vi "AMVoltsordB.vi"(8 "Min Power":dbl=10.0, 9 "Peak Power":dbl=20.0, 10 "Signal In":dbl, 11 "Linear?":bool) -> (2 "Out":dbl)   [LabVIEW 2012]
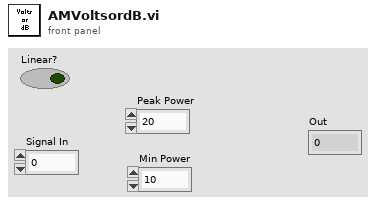
[diagram p1: front panel]
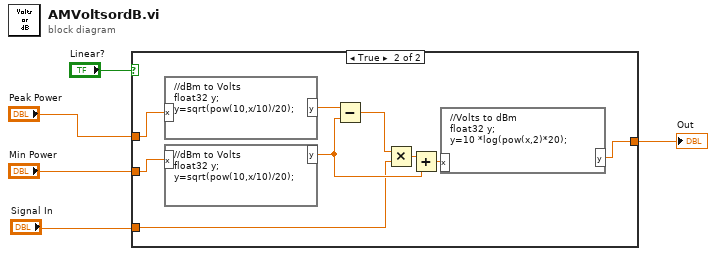
[diagram p0: block diagram]
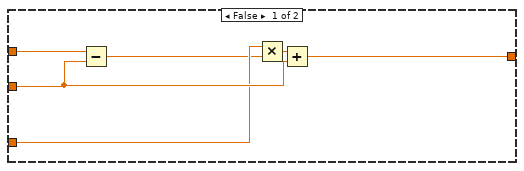
[diagram p2: hidden frame]
diagram:
  n1 = case shown="True" "Linear?" {
    tunnel: [w10 w13] -> w5
    tunnel: "Peak Power" -> [w9 w16]
    tunnel: "Min Power" -> [w8 w15]
    tunnel: "Signal In" -> [w7 w14]
    frame False {
      n2 = Subtract(x=w9, y=w8) -> (x-y=w6:dbl)
      n3 = Multiply(x=w7, y=w6) -> (x*y=w11:dbl)
      n4 = Add(x=w11, y=w8) -> (x+y=w10:dbl)
    }
    frame True {
      n5 = formula code="//dBm to Volts\nfloat32 y;\ny=sqrt(pow(10,x/10)/20);"("x"=w16) -> ("y"=w19:sgl)
      n6 = formula code="//dBm to Volts\nfloat32 y;\ny=sqrt(pow(10,x/10)/20);"("x"=w15) -> ("y"=w20:sgl)
      n7 = Subtract(x=w19, y=w20) -> (x-y=w12:sgl)
      n8 = Multiply(x=w12, y=w14) -> (x*y=w17:dbl)
      n9 = Add(x=w17, y=w20) -> (x+y=w18:dbl)
      n10 = formula code="//Volts to dBm\nfloat32 y;\ny=10 *log(pow(x,2)*20);"("x"=w18) -> ("y"=w13:sgl)
    }
  }
  "Out" <- w5
